vi "sub_device2.vi"   [LabVIEW 2017]
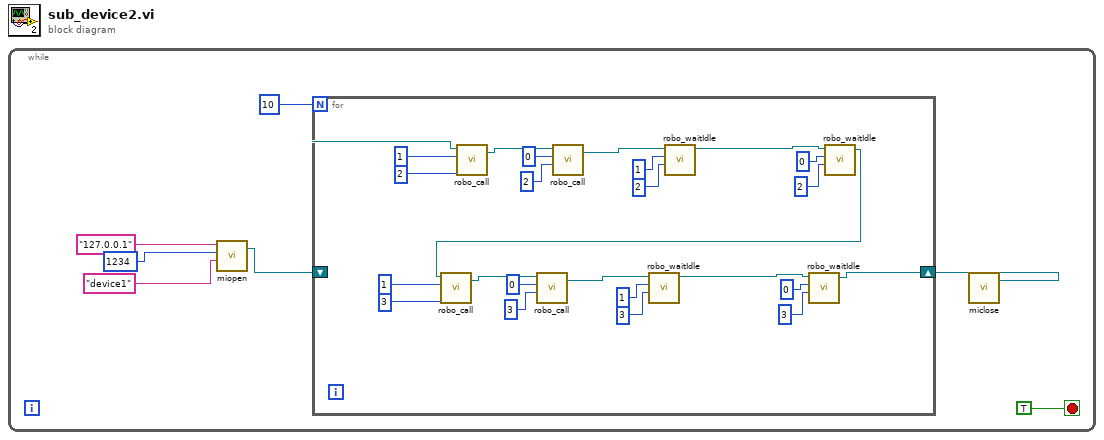
[diagram p0: block diagram]
diagram:
  n1 = while {
    stop <- TRUE stop-if-true
    n2 = call "miopen.vi"("name"="device1", "port"=u16 1234, "ip"="127.0.0.1") -> ("VISA资源名称输出"=w3:refnum<visa-resource-name>)  [unwired: 1 in, 1 out]
    n3 = for {
      N: 10 -> [_]
      shift-right: [w10] -> w7
      shift-left: w3 -> [w9]
      n4 = call "robo_call.vi"("page"=2, "ax"=1, "VISA资源名称"=w9) -> ("VISA资源名称输出"=w31:refnum<visa-resource-name>)  [unwired: 3 in, 1 out]
      n5 = call "robo_call.vi"("page"=2, "ax"=0, "VISA资源名称"=w31) -> ("VISA资源名称输出"=w23:refnum<visa-resource-name>)  [unwired: 3 in, 1 out]
      n6 = call "robo_waitIdle.vi"("VISA资源名称"=w23, "ax"=1, "page"=2) -> ("VISA资源名称输出"=w24:refnum<visa-resource-name>)  [unwired: 2 in, 2 out]
      n7 = call "robo_waitIdle.vi"("VISA资源名称"=w24, "ax"=0, "page"=2) -> ("VISA资源名称输出"=w11:refnum<visa-resource-name>)  [unwired: 2 in, 2 out]
      n8 = call "robo_call.vi"("page"=3, "ax"=1, "VISA资源名称"=w11) -> ("VISA资源名称输出"=w20:refnum<visa-resource-name>)  [unwired: 3 in, 1 out]
      n9 = call "robo_call.vi"("page"=3, "ax"=0, "VISA资源名称"=w20) -> ("VISA资源名称输出"=w12:refnum<visa-resource-name>)  [unwired: 3 in, 1 out]
      n10 = call "robo_waitIdle.vi"("VISA资源名称"=w12, "ax"=1, "page"=3) -> ("VISA资源名称输出"=w13:refnum<visa-resource-name>)  [unwired: 2 in, 2 out]
      n11 = call "robo_waitIdle.vi"("VISA资源名称"=w13, "ax"=0, "page"=3) -> ("VISA资源名称输出"=w10:refnum<visa-resource-name>)  [unwired: 2 in, 2 out]
    }
    n12 = call "miclose.vi"("VISA资源名称"=w7) -> ()  [unwired: 1 in, 1 out]
  }
